vi "Update Plot.vi"(8 "error in (no error)":errorcluster, 10 "joint positions":dbl[](array[numeric]), 11 "serial arm in":refnum<class "NI_Robotics_Serial Robot Arm.lvclass">) -> (0 "error out":errorcluster, 2 "serial arm scene":refnum<vi>, 3 "serial arm out":refnum<class "NI_Robotics_Serial Robot Arm.lvclass">)   [LabVIEW 2017, in "NI_Robotics_3DKinematics.lvlib"]
doc: "Returns a 3D scene with the 3D object that represents a robotic arm. You must use the Initialize Plot VI to initialize the 3D object before you call this VI for the first time."
uses:
  <vilib>/robotics/Kinematics/Plotting/NI_Robotics_3DKinematics.lvlib
  <vilib>/robotics/Kinematics/Robot/NI_Robotics_Serial Robot Arm.lvclass
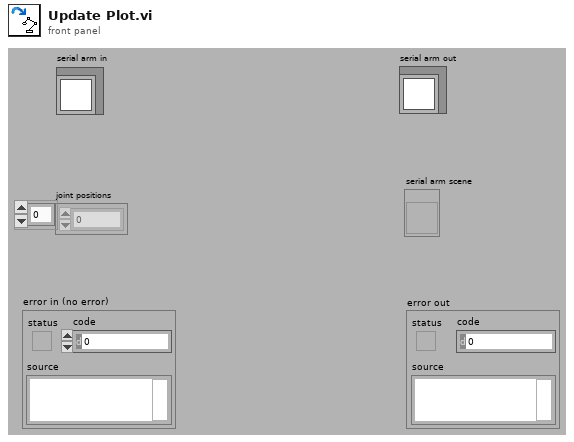
[diagram p1: front panel]
types:
  T1 = typedef "NI_Robotics_3DKinematics.lvlib/Joint Control.ctl" = cluster{"Joint Refnum":refnum<vi>, "Joint Type":T2, "Position WRT Parent":dbl[], "Rotation WRT Parent":dbl[], "Bar Refnum":refnum<vi>}
  T2 = typedef "NI_Robotics_3DKinematics.lvlib/Joint Type.ctl" = enum16{"Trans_X", "Trans_Y", "Trans_Z", "Rot_X", "Rot_Y", "Rot_Z", "None"}
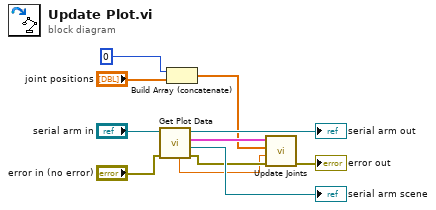
[diagram p0: block diagram]
diagram:
  n1 = call <vilib>:"Get Plot Data.vi"("error in (no error)"="error in (no error)", "NI_Robotics_Serial Robot Arm in"="serial arm in") -> ("error out"=w5:errorcluster, "Serial Arm Scene"=→"serial arm scene":refnum<vi>, "Plot Data"=w4:T1[], "NI_Robotics_Serial Robot Arm out"=→"serial arm out":refnum<class "NI_Robotics_Serial Robot Arm.lvclass">, "Scale"=w3:dbl)  [unwired: 5 in]
  n2 = Build Array (concatenate)(0 ("Slide"), "joint positions") -> (w2:dbl[])
  n3 = call <vilib>:"Update Joints.vi"("error in (no error)"=w5, "Scale (1)"=w3, "Joints"=w2, "Joint Array"=w4) -> ("error out"=→"error out":errorcluster)  [unwired: 7 in]
